vi "NXT normalize array A.vi"(1 "FB Arbiter\nVelocity":i16=4, 2 "Tug array":i16[](array[numeric])=[0]) -> (0 "Normalized\nArray":i16[](array[numeric]))   [LabVIEW 2012]
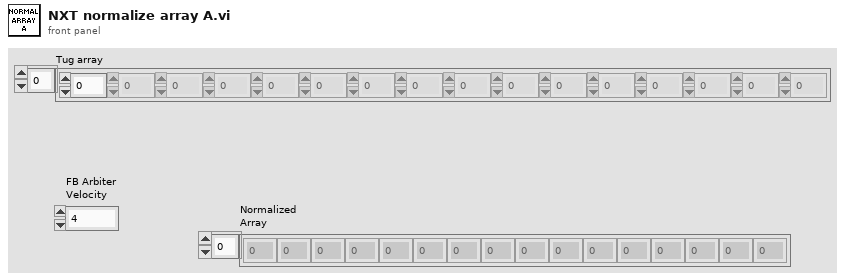
[diagram p1: front panel]
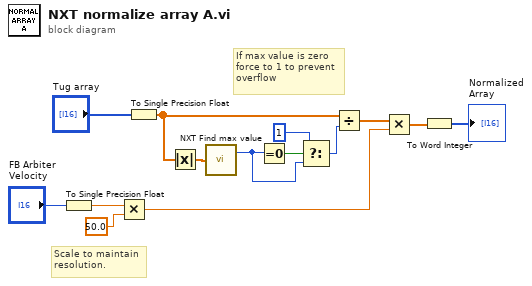
[diagram p0: block diagram]
diagram:
  # "Scale to maintain\nresolution."
  # "If max value is zero\nforce to 1 to prevent\noverflow"
  n1 = To Single Precision Float(number="FB Arbiter\nVelocity") -> (single precision float=w3:sgl)
  n2 = Multiply(x=w3, y=sgl 50.0) -> (x*y=w1:sgl)
  n3 = To Single Precision Float(number="Tug array") -> (single precision float=w14:sgl[])
  n4 = Absolute Value(x=w14) -> (abs(x)=w13:sgl[])
  n5 = call "NXT Find max value.vi"("array"=w13) -> ("Max Value"=w8:i16)  [unwired: 1 out]
  n6 = Equal To 0?(x=w8) -> (x = 0?=w9:bool)
  n7 = Select(t=i16 1, s=w9, f=w8) -> (s? t:f=w6:i16)
  n8 = Divide(x=w14, y=w6) -> (x/y=w12:sgl[])
  n9 = Multiply(x=w12, y=w1) -> (x*y=w5:sgl[])
  n10 = To Word Integer(number=w5) -> (16bit integer=→"Normalized\nArray":i16[])
